vi "Write response queue.vi"(10 "communicator":refnum<class "communicator.lvclass">, 11 "communicator message in":refnum<class "communicator message.lvclass">) -> (3 "communicator message out":refnum<class "communicator message.lvclass">)   [LabVIEW 2015, in "communicator message.lvclass"]
uses:
  communicator message.lvclass
  communicator/communicator.lvclass
  communicator message.lvclass/communicator message.ctl
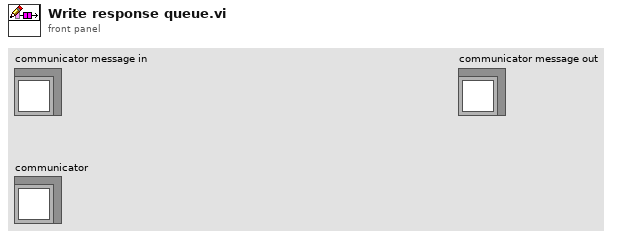
[diagram p1: front panel]
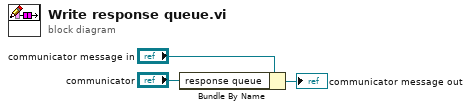
[diagram p0: block diagram]
diagram:
  n1 = Bundle By Name(cluster="communicator message in", "response queue"="communicator") -> (→"communicator message out":refnum<class "communicator message.lvclass">)
